vi "Generate Sound.vi"() -> ()   [LabVIEW 2021]
doc: "This VI illustrates how to generate and play sine, square, sawtooth and triangle waveforms. You can change the frequency and type of the waveform generated as it plays continuously."
uses:
  <vilib>/sound2/lvsound2.llb/Sampling Mode.ctl
  <vilib>/sound2/lvsound2.llb/Sound Data Format.ctl
  <vilib>/sound2/lvsound2.llb/Sound Output Set Volume (Single).vi
  <vilib>/sound2/lvsound2.llb/Sound Output Write (DBL Single).vi
  <vilib>/measure/NI_MABase.lvlib
panel:
  in  "Frequency 2":dbl=500.0
  in  "Volume":dbl(slide)=50.0 scale=0.0..100.0
  out "Generated Sound":waveform(dbl)(graph)
  in  "Frequency":dbl=500.0
  in  "Stop":bool
  in  "Device ID":u32
  # "Overview: Demonstrates the use of the Sound Functions to generate and play a sine waveform continuously.\nInstructions:\n1. Specify the Device ID.\n2. Run the VI. Waveforms are generated and sent to both the graph and your speakers.\n3. Change the Frequency and Volume of the sound.\n4. Click Stop to stop the VI."
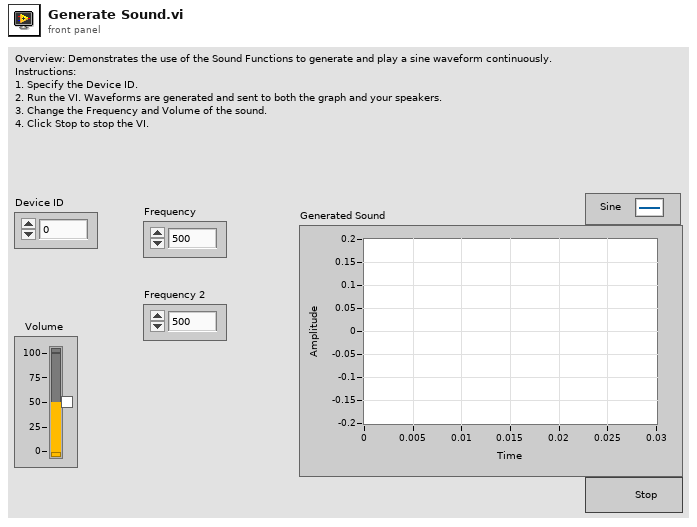
[diagram p1: front panel]
types:
  T1 = typedef "Sound Data Format.ctl" = cluster{"sample rate (S/s)":dbl, "number of channels":i32, "bits per sample":i32}
  T2 = typedef "Sampling Mode.ctl" = i32
  T3 = typedef "Sound Output Task ID.ctl" = u32
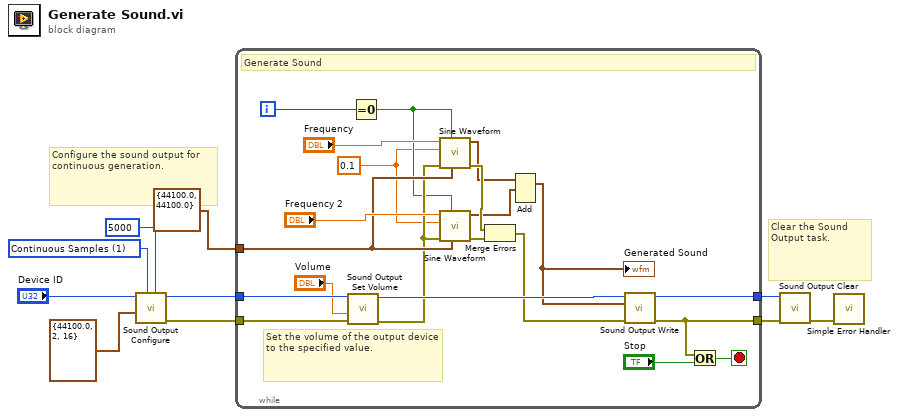
[diagram p0: block diagram]
diagram:
  w5 = T2 1 items=["Finite Samples", "Continuous Samples"] ("sample mode")
  # "Configure the sound output for continuous generation."
  # "Clear the Sound Output task."
  n1 = call <vilib>:"Sound Output Configure.vi"("number of samples/ch"=5000 ("Number of Samples/ch"), "sample mode"=w5, "sound format"=T1 {"sample rate (S/s)"=44100.0, "number of channels"=2, "bits per sample"=16} ("Sound Format"), "device ID"="Device ID") -> ("error out"=w10:errorcluster, "task ID"=w9:T3)  [unwired: 6 in]
  n2 = while {
    tunnel: w9 -> [w26]
    tunnel: [w31] -> w7
    tunnel: w10 -> [w28]
    tunnel: [w24] -> w8
    tunnel: cluster{"Fs":dbl, "#s":dbl} {"Fs"=44100.0, "#s"=44100.0} ("sampling info") -> [w21]
    i -> [w13]
    stop <- w29 stop-if-true
    w11 = 0.1 ("amplitude")
    # "Set the volume of the output device to the specified value."
    # "Generate Sound"
    n3 = call-poly <vilib>:"Sound Output Set Volume.vi"("error in (no error)"=w28, "volume"="Volume", "task ID"=w26) -> ("error out"=w20:errorcluster, "task ID out"=w27:T3)  [unwired: 7 in]
    n4 = Equal To 0?(x=w13) -> (x = 0?=w12:bool)
    n5 = call <vilib>:"Sine Waveform.vi"("sampling info"=w21, "reset signal"=w12, "error in (no error)"=w20, "amplitude"=w11, "frequency"="Frequency") -> ("error out"=w18:errorcluster, "signal out"=w16:waveform(dbl))  [unwired: 5 in]
    n6 = call <vilib>:"Sine Waveform.vi"("sampling info"=w21, "reset signal"=w12, "error in (no error)"=w20, "amplitude"=w11, "frequency"="Frequency 2") -> ("error out"=w19:errorcluster, "signal out"=w15:waveform(dbl))  [unwired: 5 in]
    n7 = Merge Errors(w18, w19) -> (w17:errorcluster)
    n8 = Add(1:w15, 2:w16) -> (0:w14:waveform(dbl))  [unwired: 1 in, 1 out]
    "Generated Sound" <- w14
    n9 = call-poly <vilib>:"Sound Output Write.vi"("error in (no error)"=w17, "data"=w14, "task ID"=w27) -> ("error out"=w24:errorcluster, "task ID out"=w31:T3)  [unwired: 7 in]
    n10 = Or(x=w24, y="Stop") -> (x .or. y?=w29:bool)
  }
  n11 = call <vilib>:"Sound Output Clear.vi"("error in (no error)"=w8, "task ID"=w7) -> ("error out"=w3:errorcluster)  [unwired: 9 in]
  n12 = call <vilib>:"Simple Error Handler.vi"("error in (no error)"=w3) -> ()  [unwired: 4 in, 5 out]
